vi "calc_pumptimemonitor.vi"(8 "error in (no error)":errorcluster, 10 "Interval (ms)":dbl, 11 "Initial timestamp":timestamp) -> (0 "error out":errorcluster, 1 "Stop?":bool, 2 "Stop time (s)":dbl, 3 "Time since start (s)":dbl)   [LabVIEW 2018]
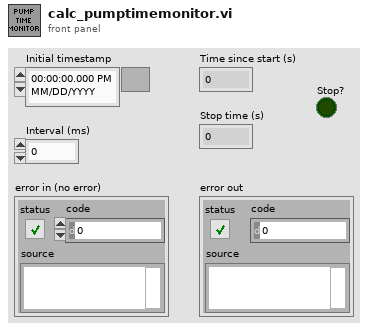
[diagram p1: front panel]
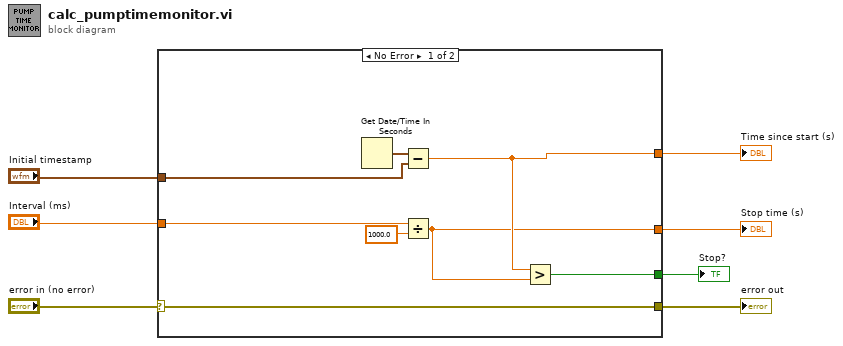
[diagram p0: block diagram]
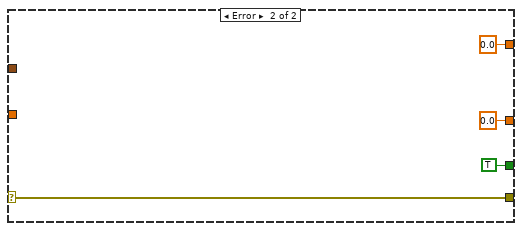
[diagram p2: hidden frame]
diagram:
  n1 = case shown="No Error" "error in (no error)" {
    selector: "error in (no error)" -> [w9 w19]
    tunnel: "Initial timestamp" -> [w13 _]
    tunnel: "Interval (ms)" -> [w12 _]
    tunnel: [w11 0.0] -> w4
    tunnel: [w10 0.0] -> w3
    tunnel: [w9 w19] -> w2
    tunnel: [w8 TRUE] -> w1
    frame No Error {
      n2 = Get Date/Time In Seconds() -> (seconds since 1Jan1904=w15:timestamp)
      n3 = Subtract(x=w15, y=w13) -> (x-y=w11:dbl)
      n4 = Divide(x=w12, y=1000.0) -> (x/y=w10:dbl)
      n5 = Greater?(x=w11, y=w10) -> (0:w8:bool)
    }
    frame Error {
    }
  }
  "error out" <- w2
  "Stop time (s)" <- w3
  "Time since start (s)" <- w4
  "Stop?" <- w1
